vi "week08_Ex02.vi"() -> ()   [LabVIEW 2017]
panel:
  in  "Money":T1(ring)=enum."KRW"
  in  "stop":bool
  out "Money USA":dbl
  in  "Money Baht":dbl
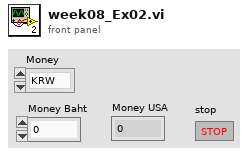
[diagram p1: front panel]
types:
  T1 = enum16{"UNKNOW", "USD", "THB", "TWD", "KRW", "JPY", "CNY", "EUR"}
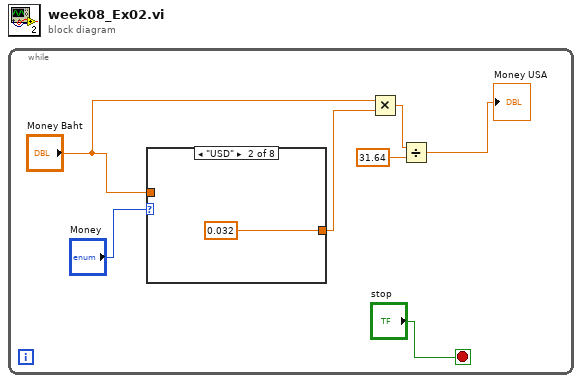
[diagram p0: block diagram]
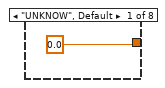
[diagram p2: hidden frame]
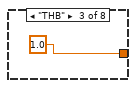
[diagram p3: hidden frame]
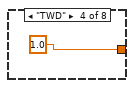
[diagram p4: hidden frame]
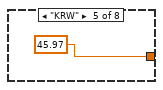
[diagram p5: hidden frame]
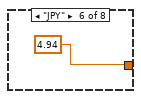
[diagram p6: hidden frame]
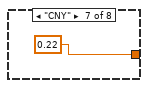
[diagram p7: hidden frame]
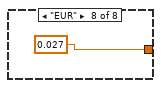
[diagram p8: hidden frame]
diagram:
  n1 = while {
    stop <- "stop" stop-if-true
    n2 = case shown="\"USD\"" "Money" {
      tunnel: "Money Baht" -> [_ _ _ _ _ _ _ _]
      tunnel: [0.0 ("y") 0.032 ("y") 1.0 ("y") 1.0 ("y") 45.97 ("y") 4.94 ("y") 0.22 ("y") 0.027 ("y")] -> w5
      frame "UNKNOW", Default {
      }
      frame "USD" {
      }
      frame "THB" {
      }
      frame "TWD" {
      }
      frame "KRW" {
      }
      frame "JPY" {
      }
      frame "CNY" {
      }
      frame "EUR" {
      }
    }
    n3 = Multiply(x="Money Baht", y=w5) -> (x*y=w4:dbl)
    n4 = Divide(x=w4, y=31.64) -> (x/y=→"Money USA":dbl)
  }
